vi "Bin move.vi"(1 "Color":i32, 2 "Array Position":cluster{"Row":i32, "Column":i32}, 3 "Chess Array":i32[][](array[numeric])=[[140, 130, 120, 110, 100, 111, 121, 131, 141], [-1, -1, -1, -1, -1, -1, -1, -1, -1], [-1, 150, -1, -1, -1, -1, -1, 151, -1], [160, -1, 161, -1, 162, -1, 163, -1, 164], [-1, -1, -1, -1, -1, -1, -1, -1, -1], [-1, -1, -1, -1, -1, -1, -1, -1, -1], [260, -1, 261, -1, 262, -1, 263, -1, 264], [-1, 250, -1, -1, -1, -1, -1, 251, -1], [-1, -1, -1, -1, -1, -1, -1, -1, -1], [240, 230, 220, 210, 200, 211, 221, 231, 241]]) -> (0 "Shuai move":cluster{i32, i32}[](array[cluster]))   [LabVIEW 2009]
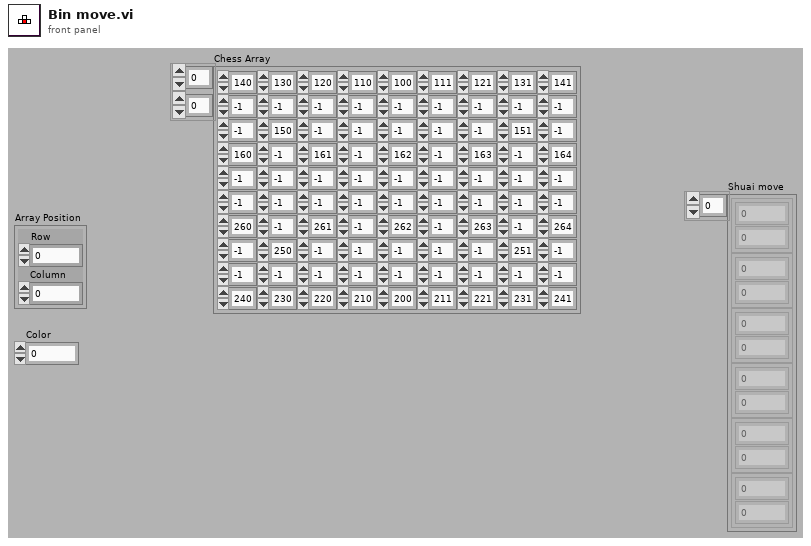
[diagram p1: front panel]
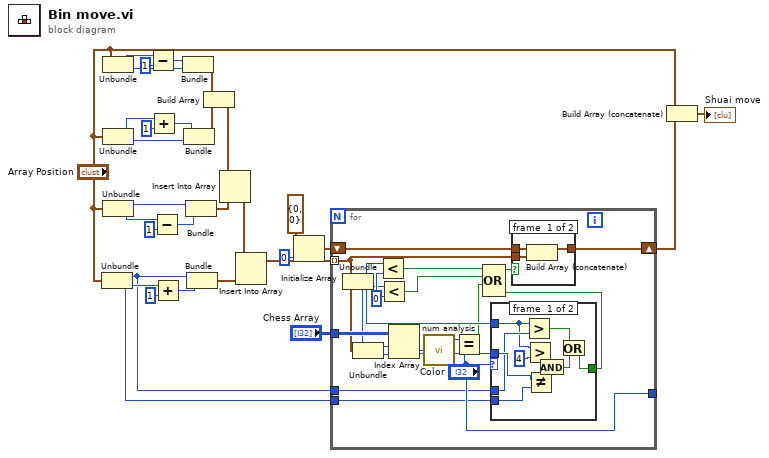
[diagram p0: block diagram]
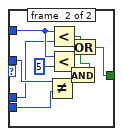
[diagram p2: hidden frame]
diagram:
  n1 = Unbundle("Array Position") -> ("Row"=w2:i32, "Column"=w5:i32)
  n2 = Unbundle("Array Position") -> ("Row"=w6:i32, "Column"=w30:i32)
  n3 = Unbundle("Array Position") -> ("Row"=w29:i32, "Column"=w26:i32)
  n4 = Unbundle("Array Position") -> ("Row"=w25:i32, "Column"=w27:i32)
  n5 = Subtract(x=w6, y=1) -> (x-y=w13:i32)
  n6 = Add(x=w29, y=1) -> (x+y=w11:i32)
  n7 = Subtract(x=w27, y=1) -> (x-y=w9:i32)
  n8 = Add(x=w5, y=1) -> (x+y=w7:i32)
  n9 = Bundle(w13, "Column"=w30) -> (w20:cluster{i32, "Column":i32})  [unwired: 1 out]
  n10 = Bundle(w11, "Column"=w26) -> (w19:cluster{i32, "Column":i32})  [unwired: 1 out]
  n11 = Bundle("Row"=w25, w9) -> (w17:cluster{"Row":i32, i32})  [unwired: 1 out]
  n12 = Bundle("Row"=w2, w7) -> (w15:cluster{"Row":i32, i32})  [unwired: 1 out]
  n13 = Build Array(w20, w19) -> (w18:cluster{i32, "Column":i32}[])
  n14 = Insert Into Array(array=w18, new element=w17) -> (w16:cluster{i32, "Column":i32}[])  [unwired: 1 in]
  n15 = Insert Into Array(array=w16, new element=w15) -> (w24:cluster{i32, "Column":i32}[])  [unwired: 1 in]
  n16 = Initialize Array(cluster{i32, i32} {0, 0} ("Output Cluster"), 0 ("Dimension Size")) -> (w23:cluster{i32, i32}[])
  n17 = for {
    tunnel: w24 -> [w38] mode=indexing
    shift-right: [w44] -> w4
    shift-left: w23 -> [w45]
    tunnel: "Chess Array" -> [w43]
    tunnel: ["Color"] -> _
    tunnel: w2 -> [w32]
    tunnel: w5 -> [w31]
    w49 = 0 ("y")
    n18 = Unbundle(w38) -> (w37:i32, "Column"=w33:i32)
    n19 = Unbundle(w38) -> (w40:i32, "Column"=w39:i32)
    n20 = Less?(x=w37, y=w49) -> (x < y?=w47:bool)
    n21 = Less?(x=w33, y=w49) -> (x < y?=w48:bool)
    n22 = Index Array(array=w43, index (row)=w40, index (col)=w39) -> (element=w42:i32)
    n23 = call "num analysis.vi"("x"=w42) -> ("Color"=w41:i32)  [unwired: 2 out]
    n24 = Equal?(x=w41, y="Color") -> (x = y?=w36:bool)
    n25 = case shown="1, Default" "Color" {
      tunnel: w37 -> [w50 w62]
      tunnel: [w53 w63] -> w35
      tunnel: w32 -> [w52 w61]
      tunnel: w33 -> [w58 w68]
      tunnel: w31 -> [w51 w60]
      frame #0 {
        n26 = Greater?(x=w50, y=w52) -> (0:w55:bool)
        n27 = Greater?(x=w50, y=4) -> (0:w57:bool)
        n28 = Not Equal?(x=w58, y=w51) -> (x != y?=w56:bool)
        n29 = And(x=w57, y=w56) -> (x .and. y?=w54:bool)
        n30 = Or(x=w55, y=w54) -> (x .or. y?=w53:bool)
      }
      frame #1 {
        n31 = Not Equal?(x=w68, y=w60) -> (x != y?=w66:bool)
        n32 = Less?(x=w62, y=w61) -> (x < y?=w64:bool)
        n33 = Less?(x=w62, y=5) -> (x < y?=w67:bool)
        n34 = And(x=w67, y=w66) -> (x .and. y?=w65:bool)
        n35 = Or(x=w64, y=w65) -> (x .or. y?=w63:bool)
      }
    }
    n36 = Compound Arithmetic op=OR(w47, w48, w36, w35) -> (w46:bool)
    n37 = case shown="False" w46 {
      tunnel: w45 -> [w72 w73]
      tunnel: [w71 w73] -> w44
      tunnel: w38 -> [w70 _]
      frame #0 {
        n38 = Build Array (concatenate)(w72, w70) -> (w71:cluster{i32, "Column":i32}[])
      }
      frame #1 {
      }
    }
  }
  n39 = Build Array (concatenate)(w4, "Array Position") -> (→"Shuai move":cluster{"Row":i32, "Column":i32}[])
